vi "getCurrent_channel.vi"(8 "error in (no error)":errorcluster, 9 "Samples":dbl=1024.0, 10 "Channel":i8, 11 "TecellaClient in":refnum<class "TecellaClient.lvclass">) -> (0 "error out":errorcluster, 2 "Currents":dbl[][](array[numeric]), 3 "TecellaClient out":refnum<class "TecellaClient.lvclass">)   [LabVIEW 2009, in "TecellaClient.lvclass"]
uses:
  TecellaClient.lvclass
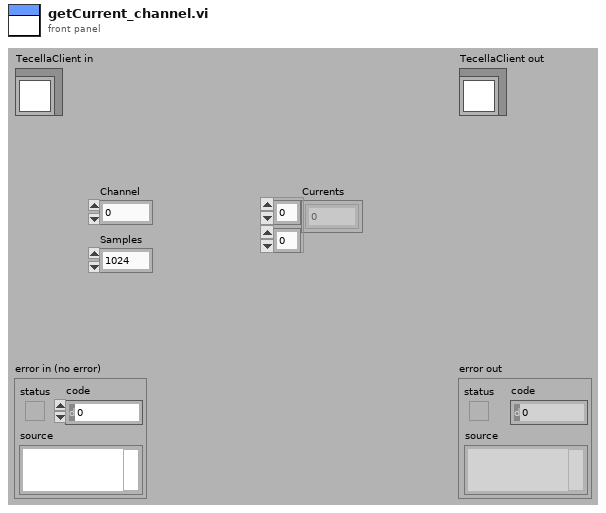
[diagram p1: front panel]
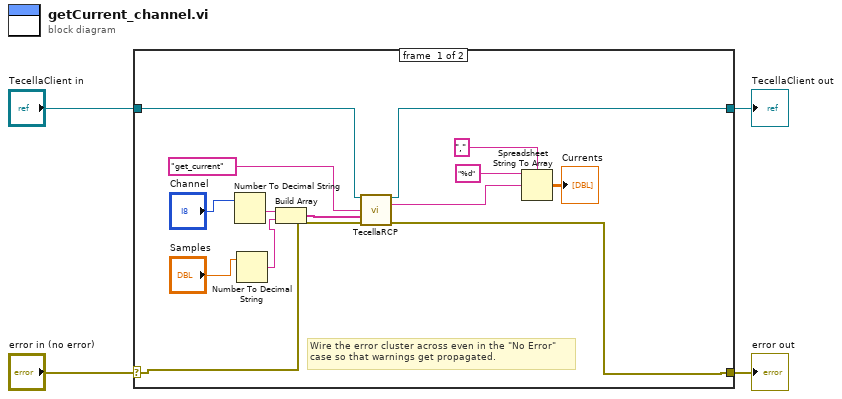
[diagram p0: block diagram]
diagram:
  n1 = case shown="No Error" "error in (no error)" {
    selector: "error in (no error)" -> [w16 w20]
    tunnel: [w7 w20] -> w3
    tunnel: [w17 w19] -> w1
    tunnel: "TecellaClient in" -> [w18 w19]
    frame #0 {
      # "Wire the error cluster across even in the \"No Error\"\ncase so that warnings get propagated."
      n2 = Number To Decimal String(number="Channel") -> (decimal integer string=w13:string)  [unwired: 1 in]
      n3 = Number To Decimal String(number="Samples") -> (decimal integer string=w5:string)  [unwired: 1 in]
      n4 = Build Array(w13, w5) -> (w14:string[])
      n5 = call-dynamic "TecellaRCP.vi"("TecellaClient in"=w18, "method"="get_current", "Args"=w14, "error in (no error)"=w16) -> ("TecellaClient out"=w17:refnum<class "TecellaClient.lvclass">, "Data Returned"=w11:string, "error out"=w7:errorcluster)  [unwired: 9 in]
      n6 = Spreadsheet String To Array(delimiter (Tab)=",", format string="%d", spreadsheet string=w11) -> (array=→"Currents":dbl[][])  [unwired: 1 in]
    }
    frame #1 {
    }
  }
  "error out" <- w3
  "TecellaClient out" <- w1
